vi "TELLC CtrlRef palette vis.vi"   [LabVIEW 2017]
uses:
  <vilib>/TELLC/Dynamic CVT API/TD Dynamic CVT DVR--ref.ctl
types:
  T1 = typedef "TD Dynamic CVT DVR--ref.ctl" = refnum<data-value>
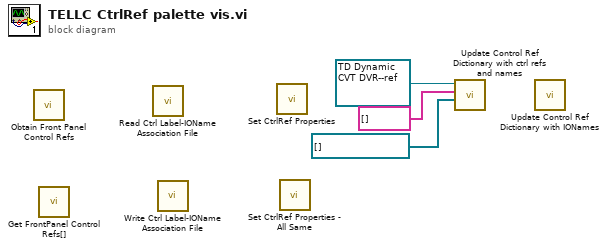
[diagram p0: block diagram]
diagram:
  n1 = call <vilib>:"Obtain Front Panel Control Refs.vi"() -> ()  [unwired: 9 in, 3 out]
  n2 = call <vilib>:"Get FrontPanel Control Refs[].vi"() -> ()  [unwired: 9 in, 3 out]
  n3 = call <vilib>:"Read Ctrl Label-IOName Association File.vi"() -> ()  [unwired: 9 in, 3 out]
  n4 = call <vilib>:"Write Ctrl Label-IOName Association File.vi"() -> ()  [unwired: 10 in, 2 out]
  n5 = call <vilib>:"Set CtrlRef Properties.vi"() -> ()  [unwired: 8 in, 3 out]
  n6 = call <vilib>:"Set CtrlRef Properties - All Same.vi"() -> ()  [unwired: 8 in, 3 out]
  n7 = call <vilib>:"Update Control Ref Dictionary with ctrl refs and names.vi"("Ctrl Refs"=refnum<vi>[] [], "Names"=string[] [], "CtrlRef Dict in"=T1 refnum) -> ()  [unwired: 7 in, 2 out]
  n8 = call <vilib>:"Update Control Ref Dictionary with IONames.vi"() -> ()  [unwired: 7 in, 5 out]
